vi "destination reached.vi"(8 "error in (no error)":errorcluster, 10 "destination":T1, 11 "current_path":T1[](array[typedef])) -> (0 "error out":errorcluster, 3 "T = destination has been reached":bool)   [LabVIEW 2021, in "Project Euler.lvlib"]
uses:
  Project Euler.lvlib
  lattice_path_node.ctl
  lattice_path_direction.ctl
panel:
  out "last (most recent) node of path":T1
  # "Development\ncontrols/indicators useful for development and testing, but which are not outputs of the VI"
  # "Input\nInputs to the VI"
  # "Output\nOutputs of the VI"
  # "Description\n\nBlank VI with error handling case. \n\nSummarize the use of this VI in this space."
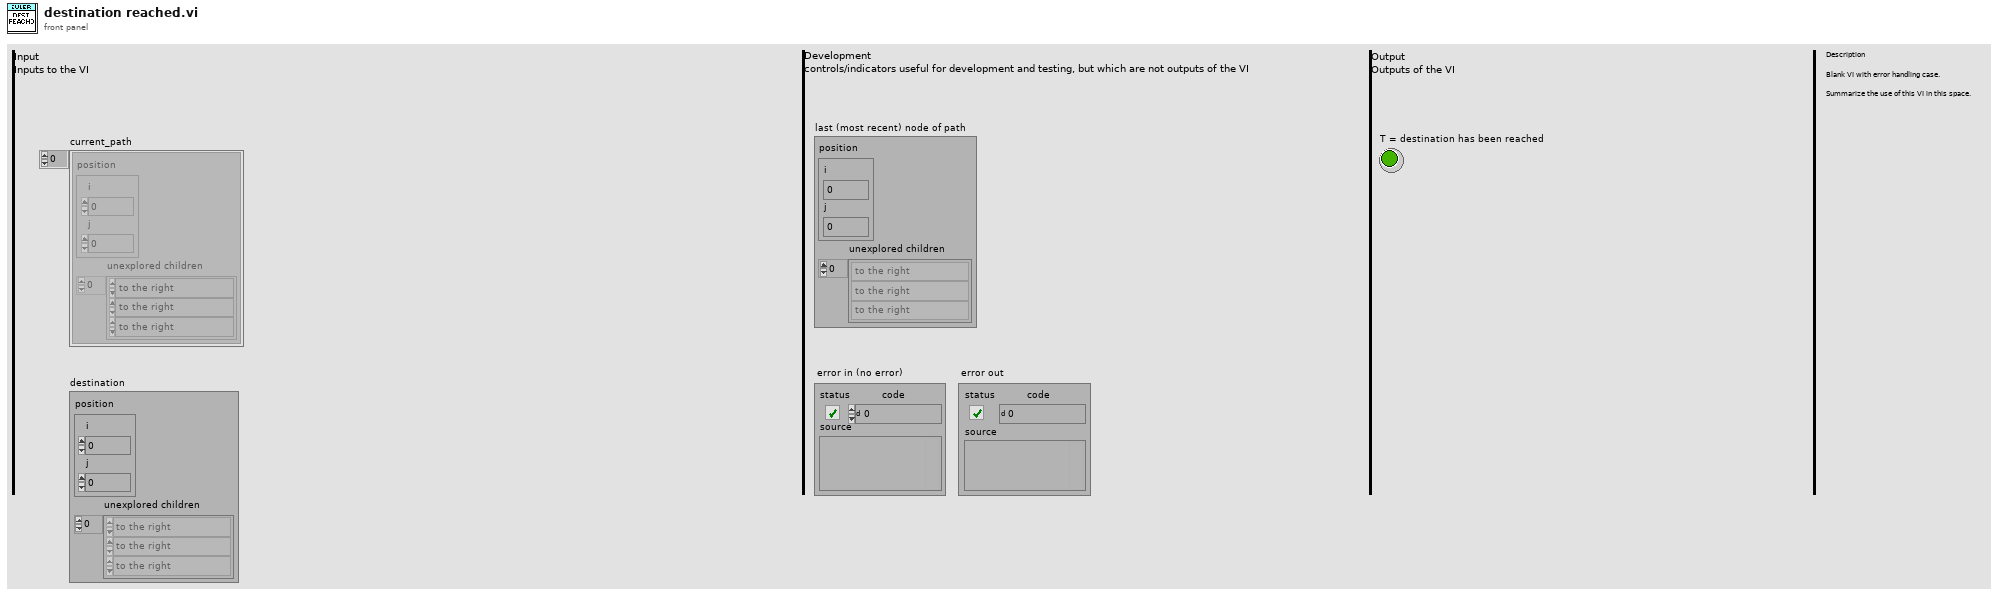
[diagram p1: front panel]
types:
  T1 = typedef "Project Euler.lvlib/lattice_path_node.ctl" = cluster{"position":cluster{"i":i32, "j":i32}, "unexplored children":T2[]}
  T2 = typedef "Project Euler.lvlib/lattice_path_direction.ctl" = enum16{"to the right", "downwards"}
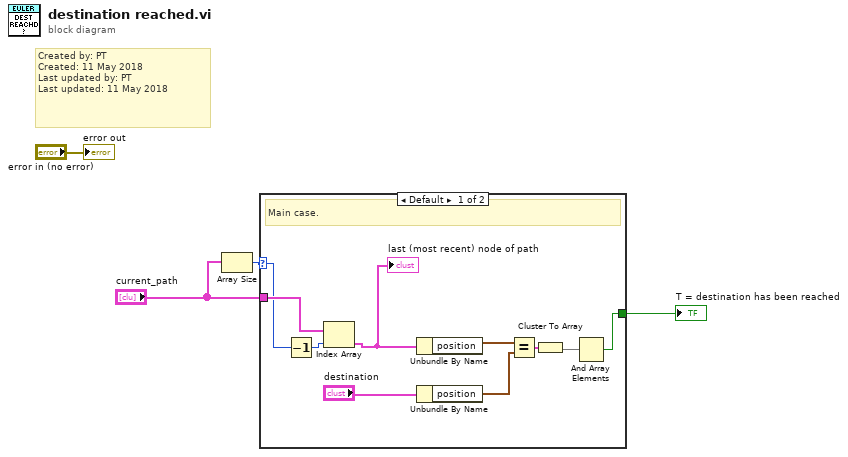
[diagram p0: block diagram]
diagram:
  # "Created by: PT\nCreated: 11 May 2018\nLast updated by: PT\nLast updated: 11 May 2018"
  n1 = Array Size(array="current_path") -> (size(s)=w2:i32)
  n2 = case shown="Default" w2 {
    selector: w2 -> [w13 _]
    tunnel: [w5 _] -> w3
    tunnel: "current_path" -> [w14 _]
    frame Default {
      # "Main case."
      n3 = Decrement(x=w13) -> (x-1=w12:i32)
      n4 = Index Array(array=w14, index=w12) -> (element=w10:T1)
      "last (most recent) node of path" <- w10
      n5 = Unbundle By Name(w10) -> ("position"=w9:cluster{"i":i32, "j":i32})
      n6 = Unbundle By Name("destination") -> ("position"=w8:cluster{"i":i32, "j":i32})
      n7 = Equal?(x=w9, y=w8) -> (x = y?=w7:cluster{"i":bool, "j":bool})
      n8 = Cluster To Array(cluster=w7) -> (array=w6:bool[])
      n9 = And Array Elements(Boolean array=w6) -> (logical AND=w5:bool)
    }
    frame 0 {
      # "Empty current path"
    }
  }
  "T = destination has been reached" <- w3
  "error out" <- "error in (no error)"
